vi "Save Config File.vi"(8 "error in (no error)":errorcluster, 10 "file path":path, 11 "queue in":T1) -> (0 "error out":errorcluster, 2 "file path out":path, 3 "queue out":T1)   [LabVIEW 2010, in "NI_LVConfig.lvlib"]
uses:
  NI_LVConfig.lvlib
  Config Queue.ctl
  Config Data.ctl
  Section.ctl
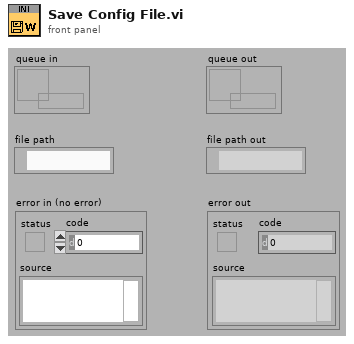
[diagram p1: front panel]
types:
  T1 = typedef "NI_LVConfig.lvlib/Config Queue.ctl" = refnum<queue>
  T2 = enum16{"open", "replace", "create", "open or create", "replace or create", "replace or create with confirmation"}
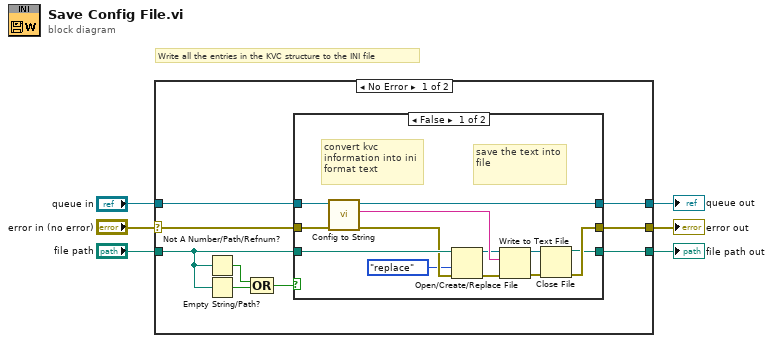
[diagram p0: block diagram]
diagram:
  # "Write all the entries in the KVC structure to the INI file"
  n1 = case shown="No Error" "error in (no error)" {
    selector: "error in (no error)" -> [w8 w34]
    tunnel: [w15 w34] -> w5
    tunnel: [w14 w33] -> w3
    tunnel: "queue in" -> [w9 w33]
    tunnel: "file path" -> [w10 w32]
    tunnel: [w7 w32] -> w1
    frame No Error {
      n2 = Not A Number/Path/Refnum?(number/path/refnum=w10) -> (NaN/Path/Refnum?=w13:bool)
      n3 = Empty String/Path?(string/path=w10) -> (empty?=w12:bool)
      n4 = Compound Arithmetic op=OR(w13, w12) -> (w11:bool)
      n5 = case shown="False" w11 {
        tunnel: [w26 w31] -> w15
        tunnel: w8 -> [w22 w31]
        tunnel: w10 -> [w23 w29]
        tunnel: w9 -> [w24 w30]
        tunnel: [w17 w30] -> w14
        tunnel: [w16 w29] -> w7
        frame False {
          # "save the text into file"
          # "convert kvc information into ini format text"
          n6 = call "Config to String.vi"("error in (no error)"=w22, "queue in"=w24) -> ("error out"=w21:errorcluster, "String"=w25:string, "queue out"=w17:T1)  [unwired: 7 out]
          n7 = Open/Create/Replace File(file path (use dialog)=w23, error in=w21, operation (0:open)=T2."replace") -> (refnum out=w19:refnum<file>, error out=w18:errorcluster)  [unwired: 4 out]
          n8 = Write to Text File(file (use dialog)=w19, text=w25, error in=w18) -> (refnum out=w28:refnum<file>, error out=w27:errorcluster)  [unwired: 2 out]
          n9 = Close File(refnum=w28, error in=w27) -> (path=w16:path, error out=w26:errorcluster)
        }
        frame True {
        }
      }
    }
    frame Error {
    }
  }
  "error out" <- w5
  "queue out" <- w3
  "file path out" <- w1
